vi "InTake GetValues.vi"(1 "InTake Global Data In":T1) -> (0 "InTake Global Data Out":T1)   [LabVIEW 2013]
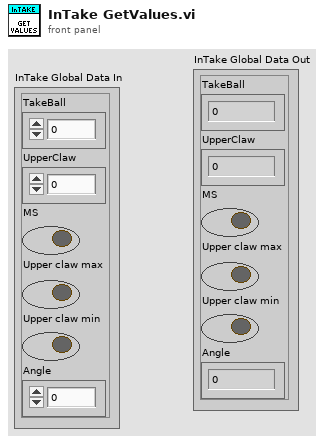
[diagram p1: front panel]
types:
  T1 = cluster{"TakeBall":dbl, "UpperClaw":dbl, "MS":bool, "Upper claw max":bool, "Upper claw min":bool, "Angle":dbl}
  T2 = typedef "WPI_DigitalInputDevRef.ctl" = cluster{"DevStatus":errorcluster, "DIO Channel":T3, "Digital Module":T4}
  T3 = typedef "FPGA_DIOChannel.ctl" = enum8{"DIO 1", "DIO 2", "DIO 3", "DIO 4", "DIO 5", "DIO 6", "DIO 7", "DIO 8", "DIO 9", "DIO 10", "DIO 11", "DIO 12", "DIO 13", "DIO 14", "Invalid"}
  T4 = typedef "FPGA_TypedefDigitalModule.ctl" = enum16{"Digital Module 1", "Digital Module 2"}
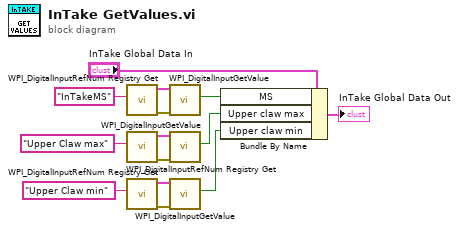
[diagram p0: block diagram]
diagram:
  n1 = call <vilib>:"WPI_DigitalInputRefNum Registry Get.vi"("refnum name"="InTakeMS") -> ("error out"=w11:errorcluster, "DigitalInputDevRef"=w12:T2)  [unwired: 9 in]
  n2 = call <vilib>:"WPI_DigitalInputRefNum Registry Get.vi"("refnum name"="Upper Claw max") -> ("error out"=w8:errorcluster, "DigitalInputDevRef"=w7:T2)  [unwired: 9 in]
  n3 = call <vilib>:"WPI_DigitalInputRefNum Registry Get.vi"("refnum name"="Upper Claw min") -> ("error out"=w5:errorcluster, "DigitalInputDevRef"=w6:T2)  [unwired: 9 in]
  n4 = call <vilib>:"WPI_DigitalInputGetValue.vi"("error in (no error)"=w11, "DigitalInputDevRef"=w12) -> ("Value"=w9:bool)  [unwired: 7 in, 2 out]
  n5 = call <vilib>:"WPI_DigitalInputGetValue.vi"("error in (no error)"=w8, "DigitalInputDevRef"=w7) -> ("Value"=w2:bool)  [unwired: 7 in, 2 out]
  n6 = call <vilib>:"WPI_DigitalInputGetValue.vi"("error in (no error)"=w5, "DigitalInputDevRef"=w6) -> ("Value"=w1:bool)  [unwired: 7 in, 2 out]
  n7 = Bundle By Name(cluster="InTake Global Data In", "MS"=w9, "Upper claw max"=w2, "Upper claw min"=w1) -> (→"InTake Global Data Out":T1)
